vi "GetFrames.vi"(8 "error in (no error)":errorcluster, 11 "Device Item Ref in":T2 format="%.0x") -> (0 "error out":errorcluster, 1 "Tx Frames":T1[](array[typedef]), 2 "Rx Frames":T1[](array[typedef]), 3 "Device Item Ref out":T2 format="%.0x")   [LabVIEW 2018, in "CAN Gateway System Explorer.lvlib"]
uses:
  CAN Gateway System Explorer.lvlib
  <vilib>/NI Veristand/Custom Device API/Custom Device Item Ref.ctl
  Types/FramesCluster.ctl
  Shared/Constants.vi
  <vilib>/NI Veristand/Custom Device API/Get Item Property (String).vi
  <resource>/objmgr/xnet.rc
  Shared/CAN Gateway Shared.lvlib
  <vilib>/NI Veristand/Custom Device API/Custom Device API.lvlib
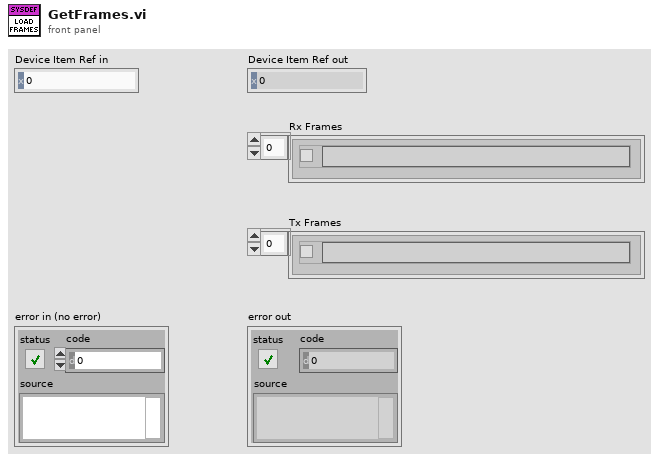
[diagram p1: front panel]
types:
  T1 = typedef "CAN Gateway System Explorer.lvlib/FramesCluster.ctl" = cluster{"Frame":string, "Fault":bool}
  T2 = typedef "Custom Device API.lvlib/Custom Device Item Ref.ctl" = u64
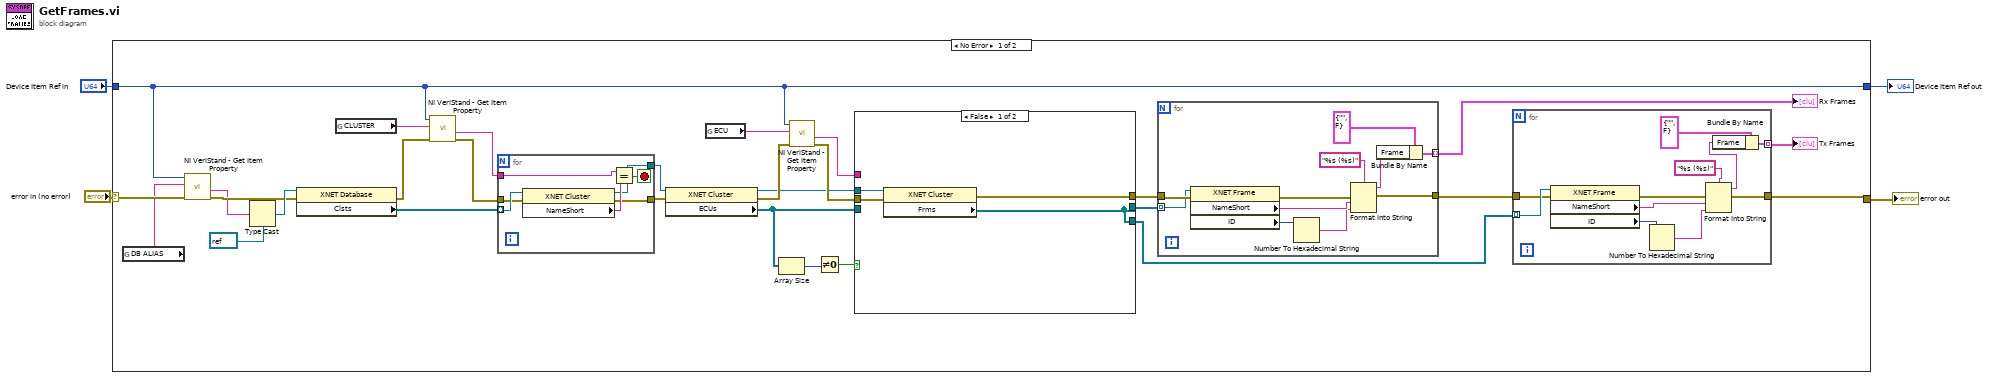
[diagram p0: block diagram]
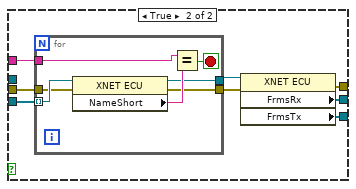
[diagram p2: hidden frame]
diagram:
  n1 = case shown="No Error" "error in (no error)" {
    selector: "error in (no error)" -> [w31 w83]
    tunnel: "Device Item Ref in" -> [w14 w82]
    tunnel: [w14 w82] -> w2
    tunnel: [w25 w83] -> w1
    frame No Error {
      n2 = global read "Constants.vi" "DB ALIAS"() -> (w22:string)
      n3 = call-poly <vilib>:"NI VeriStand - Get Item Property.vi"("error in (no error)"=w31, "Property Name"=w22, "Item Ref in"=w14) -> ("error out"=w29:errorcluster, "Value"=w18:string)  [unwired: 5 in, 2 out]
      n4 = Type Cast(type=refnum<k21> refnum ("XNET Database"), x=w18) -> (*(type *) &x=w30:refnum<k21>)
      n5 = property class="XNET Database"(reference=w30, error in=w29) -> (error out=w15:errorcluster, "Clsts"=w12:refnum<k21>[])  [unwired: 1 out]
      n6 = global read "Constants.vi" "CLUSTER"() -> (w16:string)
      n7 = call-poly <vilib>:"NI VeriStand - Get Item Property.vi"("error in (no error)"=w15, "Property Name"=w16, "Item Ref in"=w14) -> ("error out"=w13:errorcluster, "Value"=w11:string)  [unwired: 5 in, 2 out]
      n8 = for {
        tunnel: w12 -> [w59] mode=indexing
        tunnel: w13 -> [w58]
        tunnel: w11 -> [w54]
        tunnel: [w56] -> w10
        tunnel: [w55] -> w9
        stop <- w53 stop-if-true
        n9 = property class="XNET Cluster"(reference=w59, error in=w58) -> (reference out=w56:refnum<k21>, error out=w55:errorcluster, "NameShort"=w57:string)
        n10 = Equal?(x=w54, y=w57) -> (x = y?=w53:bool)
      }
      n11 = property class="XNET Cluster"(reference=w10, error in=w9) -> (reference out=w5:refnum<k21>, error out=w21:errorcluster, "ECUs"=w8:refnum<k21>[])
      n12 = global read "Constants.vi" "ECU"() -> (w20:string)
      n13 = Array Size(array=w8) -> (size(s)=w6:i32)
      n14 = call-poly <vilib>:"NI VeriStand - Get Item Property.vi"("error in (no error)"=w21, "Property Name"=w20, "Item Ref in"=w14) -> ("error out"=w19:errorcluster, "Value"=w17:string)  [unwired: 5 in, 2 out]
      n15 = Not Equal To 0?(x=w6) -> (x != 0?=w7:bool)
      n16 = case shown="False" w7 {
        tunnel: [w35 w45] -> w32
        tunnel: [w36 w44] -> w28
        tunnel: [w36 w43] -> w27
        tunnel: w8 -> [_ w42]
        tunnel: w19 -> [w37 w41]
        tunnel: w17 -> [_ w38]
        tunnel: w5 -> [w34 _]
        frame False {
          n17 = property class="XNET Cluster"(reference=w34, error in=w37) -> (error out=w35:errorcluster, "Frms"=w36:refnum<k21>[])  [unwired: 1 out]
        }
        frame True {
          n18 = for {
            tunnel: w42 -> [w52] mode=indexing
            tunnel: w41 -> [w51]
            tunnel: w38 -> [w47]
            tunnel: [w49] -> w39
            tunnel: [w48] -> w40
            stop <- w46 stop-if-true
            n19 = property class="XNET ECU"(reference=w52, error in=w51) -> (reference out=w49:refnum<k21>, error out=w48:errorcluster, "NameShort"=w50:string)
            n20 = Equal?(x=w47, y=w50) -> (x = y?=w46:bool)
          }
          n21 = property class="XNET ECU"(reference=w39, error in=w40) -> (error out=w45:errorcluster, "FrmsRx"=w44:refnum<k21>[], "FrmsTx"=w43:refnum<k21>[])  [unwired: 1 out]
        }
      }
      n22 = for {
        tunnel: w32 -> [w81]
        tunnel: [w75] -> w26
        tunnel: w28 -> [w74] mode=indexing
        tunnel: [w72] -> w24 mode=indexing
        n23 = property class="XNET Frame"(reference=w74, error in=w81) -> (error out=w77:errorcluster, "NameShort"=w79:string, "ID"=w80:u32)  [unwired: 1 out]
        n24 = Number To Hexadecimal String(2:w80) -> (0:w78:string)  [unwired: 1 in]
        n25 = Format Into String(format string="%s (%s)", error in=w77, w79, w78) -> (resulting string=w71:string, error out=w75:errorcluster)  [unwired: 1 in]
        n26 = Bundle By Name(cluster=T1 {"Frame"="", "Fault"=FALSE} ("Frame"), "Frame"=w71) -> (w72:T1)
      }
      "Rx Frames" <- w24
      n27 = for {
        tunnel: [w66] -> w25
        tunnel: w27 -> [w65] mode=indexing
        tunnel: w26 -> [w64]
        tunnel: [w62] -> w23 mode=indexing
        n28 = property class="XNET Frame"(reference=w65, error in=w64) -> (error out=w67:errorcluster, "NameShort"=w69:string, "ID"=w70:u32)  [unwired: 1 out]
        n29 = Number To Hexadecimal String(2:w70) -> (0:w68:string)  [unwired: 1 in]
        n30 = Format Into String(format string="%s (%s)", error in=w67, w69, w68) -> (resulting string=w60:string, error out=w66:errorcluster)  [unwired: 1 in]
        n31 = Bundle By Name(cluster=T1 {"Frame"="", "Fault"=FALSE} ("Frame"), "Frame"=w60) -> (w62:T1)
      }
      "Tx Frames" <- w23
    }
    frame Error {
    }
  }
  "error out" <- w1
  "Device Item Ref out" <- w2
